vi "CreateIndicator.vi"(8 "error in (no error)":errorcluster, 11 "BaseAccessorScripter in":refnum<class "BaseAccessorScripter.lvclass">) -> (0 "error out":errorcluster, 2 "New Control Ref":refnum<vi>, 3 "BaseAccessorScripter out":refnum<class "BaseAccessorScripter.lvclass">)   [LabVIEW 2021, in "MemberVICreation.lvlib" / "BaseAccessorScripter.lvclass"]
uses:
  <resource>/Framework/Providers/LVClassLibrary/NewAccessors/BaseAccessorScripter/BaseAccessorScripter.lvclass
  <resource>/Framework/Providers/LVClassLibrary/NewAccessors/BaseAccessorScripter/BaseAccessorScripter.lvclass/BaseAccessorScripter.ctl
  <resource>/Framework/Providers/LVClassLibrary/NewAccessors/MemberVICreation.lvlib
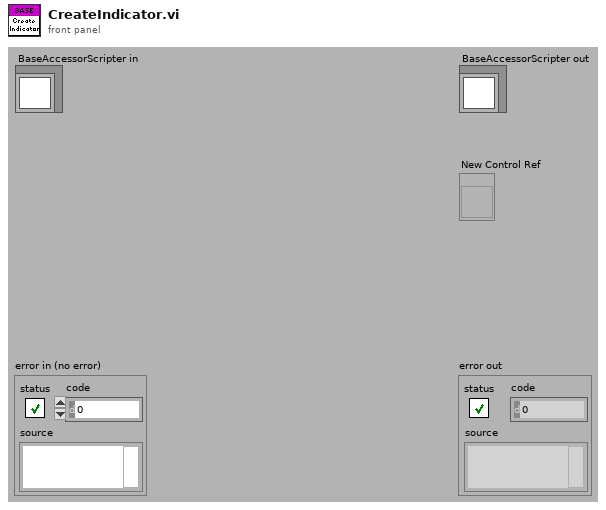
[diagram p1: front panel]
types:
  T1 = typedef "LVPositionTypeDef.ctl" = cluster{"Left":i32, "Top":i32}
  T2 = typedef "LVRectTypeDef.ctl" = cluster{"left":i16, "top":i16, "right":i16, "bottom":i16}
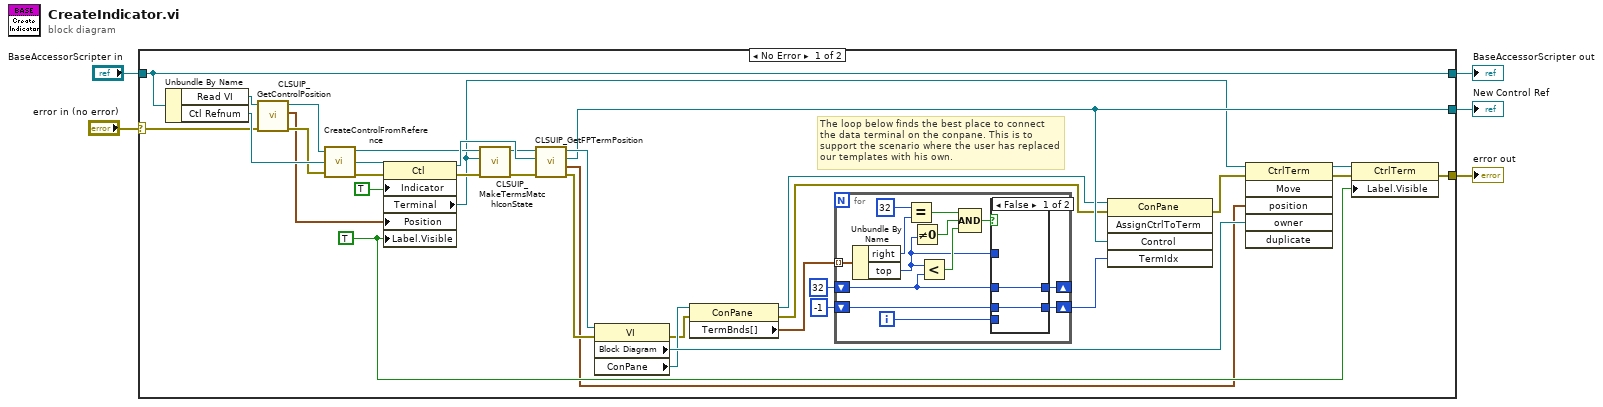
[diagram p0: block diagram]
diagram:
  n1 = case shown="No Error" "error in (no error)" {
    selector: "error in (no error)" -> [w34 w58]
    tunnel: [w19 w58] -> w1
    tunnel: [w31 w57] -> w3
    tunnel: "BaseAccessorScripter in" -> [w31 w57]
    tunnel: [w16 _] -> w2
    frame No Error {
      w17 = TRUE ("Label.Visible")
      # "The loop below finds the best place to connect the data terminal on the conpane. This is to support the scenario where the user has replaced our templates with his own."
      n2 = Unbundle By Name(w31) -> ("Read VI"=w33:refnum<vi>, "Ctl Refnum"=w39:refnum<vi>)
      n3 = call <resource>:"CLSUIP_GetControlPosition.vi"("error in (no error)"=w34, "VI Refnum"=w33) -> ("error out"=w35:errorcluster, "Position"=w26:T1, "VI Refnum out"=w32:refnum<vi>)  [unwired: 7 out]
      n4 = call <resource>:"CreateControlFromReference.vi"("error in (no error)"=w35, "Src CtlRef"=w39, "VI Refnum"=w32) -> ("error out"=w29:errorcluster, "New Object Ref"=w30:refnum<vi>, "VI Refnum out"=w23:refnum<vi>)
      n5 = property class="Ctl"(reference=w30, error in=w29, "Indicator"=TRUE, "Position"=w26, "Label.Visible"=w17) -> (reference out=w27:refnum<vi>, error out=w24:errorcluster, "Terminal"=w14:refnum<vi>)
      n6 = call <resource>:"CLSUIP_MakeTermsMatchIconState.vi"("error in (no error)"=w24, "Terminal"=w14, "VI Refnum"=w23) -> ("error out"=w21:errorcluster, "VI Refnum out"=w22:refnum<vi>)  [unwired: 7 out]
      n7 = call <resource>:"CLSUIP_GetFPTermPosition.vi"("error in (no error)"=w21, "Control Ref"=w27, "VI Refnum"=w22) -> ("error out"=w28:errorcluster, "Position"=w15:cluster{"Left":i32, "Top":i32}, "Control Ref out"=w16:refnum<vi>, "VI Refnum out"=w25:refnum<vi>)  [unwired: 5 out]
      n8 = property class="VI"(reference=w25, error in=w28) -> (error out=w12:errorcluster, "Block Diagram"=w37:refnum<vi>, "ConPane"=w13:refnum<vi>)  [unwired: 1 out]
      n9 = property class="ConPane"(reference=w13, error in=w12) -> (reference out=w7:refnum<vi>, error out=w6:errorcluster, "TermBnds[]"=w9:T2[])
      n10 = for {
        tunnel: w9 -> [w42] mode=indexing
        shift-right: [w43] -> _
        shift-left: i16 32 -> [w47]
        shift-right: [w45] -> w8
        shift-left: -1 -> [w46]
        i -> [w44]
        n11 = Unbundle By Name(w42) -> ("right"=w41:i16, "top"=w48:i16)
        n12 = Equal?(x=i16 32, y=w41) -> (x = y?=w52:bool)
        n13 = Not Equal To 0?(x=w48) -> (x != 0?=w51:bool)
        n14 = Less?(x=w48, y=w47) -> (x < y?=w50:bool)
        n15 = Compound Arithmetic op=AND(w52, w51, w50) -> (w49:bool)
        n16 = case shown="False" w49 {
          tunnel: w48 -> [_ w55]
          tunnel: w47 -> [w54 _]
          tunnel: w46 -> [w53 _]
          tunnel: [w53 w56] -> w45
          tunnel: w44 -> [_ w56]
          tunnel: [w54 w55] -> w43
          frame False {
          }
          frame True {
          }
        }
      }
      n17 = invoke class="ConPane" method="AssignCtrlToTerm"(reference=w7, error in=w6, "Control"=w16, "TermIdx"=w8) -> (error out=w36:errorcluster)  [unwired: 1 in, 4 out]
      n18 = invoke class="CtrlTerm" method="Move"(reference=w14, error in=w36, "position"=w15, "owner"=w37) -> (reference out=w18:refnum<vi>, error out=w20:errorcluster)  [unwired: 2 in, 4 out]
      n19 = property class="CtrlTerm"(reference=w18, error in=w20, "Label.Visible"=w17) -> (error out=w19:errorcluster)  [unwired: 1 out]
    }
    frame Error {
    }
  }
  "error out" <- w1
  "BaseAccessorScripter out" <- w3
  "New Control Ref" <- w2
